vi "myRIO_BRig_RT_dataAnalog_iEvent.vi"() -> (2 "output_iEvent":i32)   [LabVIEW 2014]
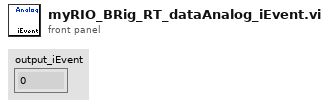
[diagram p1: front panel]
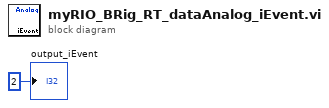
[diagram p0: block diagram]
diagram:
  "output_iEvent" <- 2 ("output_iBlock")
